vi "deinit shm info.vi"(8 "error in (no error)":errorcluster, 11 "Shared Memory runtime in":refnum<class "Shared Memory runtime.lvclass">) -> (0 "error out":errorcluster, 3 "Shared Memory runtime out":refnum<class "Shared Memory runtime.lvclass">)   [LabVIEW 2013, in "Shared Memory runtime.lvclass"]
uses:
  Shared Memory runtime.lvclass
  Shared Memory runtime.lvclass/Shared Memory runtime.ctl
  Read shm info.vi
  <vilib>/NI/Shared Memory Library/Classes/Shared Memory/Shared Memory.lvclass
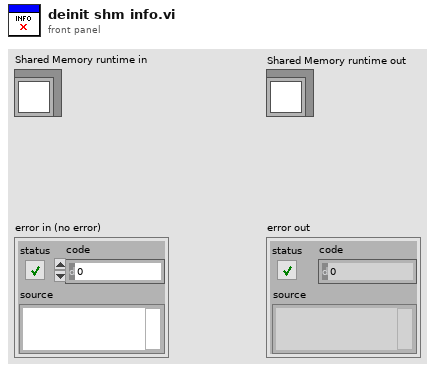
[diagram p1: front panel]
types:
  T1 = typedef "Shared Memory runtime.lvclass/shm info.ctl" = cluster{"shared memory":T2, "shm info ptrs":T3, "created?":bool}
  T2 = typedef "Shared Memory.lvlib/Shared Memory.lvclass/reference.ctl" = refnum<data-value>
  T3 = typedef "Shared Memory runtime.lvclass/shm info ptrs.ctl" = cluster{"rev_major_ptr":u64, "rev_minor_ptr":u64}
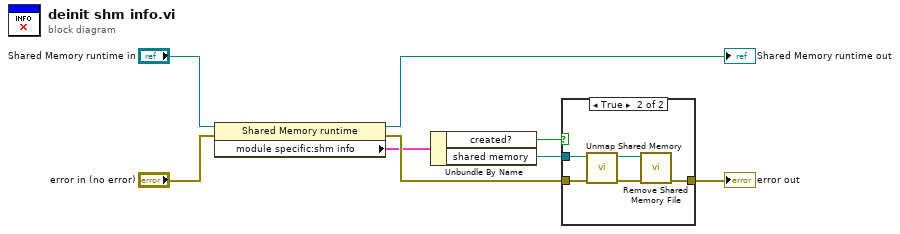
[diagram p0: block diagram]
diagram:
  n1 = property class="Shared Memory runtime"(reference="Shared Memory runtime in", error in="error in (no error)") -> (reference out=→"Shared Memory runtime out":refnum<class "Shared Memory runtime.lvclass">, error out=w4:errorcluster, "module specific:shm info"=w2:T1)
  n2 = Unbundle By Name(w2) -> ("created?"=w1:bool, "shared memory"=w5:T2)
  n3 = case shown="True" w1 {
    tunnel: w5 -> [_ w12]
    tunnel: w4 -> [w9 w11]
    tunnel: [w9 w10] -> w3
    frame False {
    }
    frame True {
      n4 = call <vilib>:"Unmap Shared Memory.vi"("error in (no error)"=w11, "shared memory in"=w12) -> ("error out"=w13:errorcluster, "shared memory out"=w14:T2)  [unwired: 8 in]
      n5 = call <vilib>:"Remove Shared Memory File.vi"("error in (no error)"=w13, "shared memory in"=w14) -> ("error out"=w10:errorcluster)  [unwired: 8 in, 1 out]
    }
  }
  "error out" <- w3
